vi "pcfs_dither_loop_wait_for_fifo_loop.vi"(8 "error in (no error)":errorcluster, 11 "pcfs in":refnum<class "pcfs.lvclass">) -> (0 "error out":errorcluster, 3 "pcfs out":refnum<class "pcfs.lvclass">)   [LabVIEW 2015, in "pcfs.lvclass"]
uses:
  pcfs.lvclass
  pcfs.lvclass/pcfs.ctl
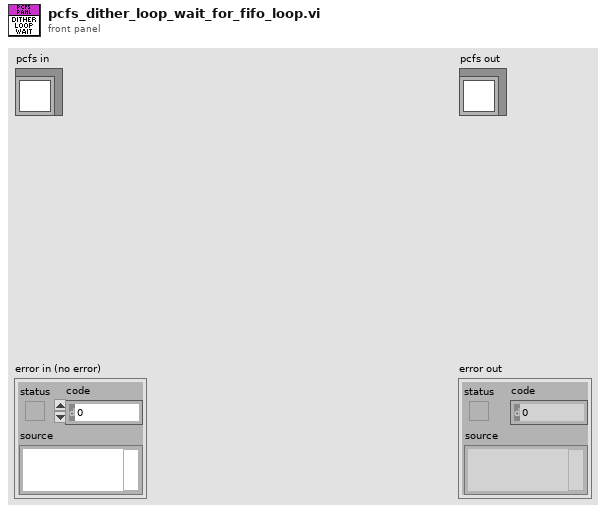
[diagram p1: front panel]
types:
  T1 = typedef "Rendezvous RefNum" = refnum<k1>
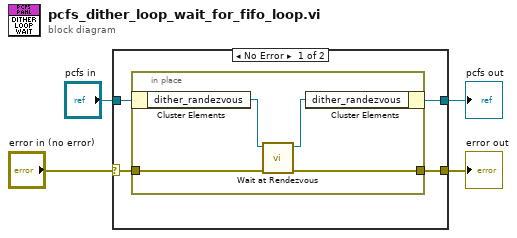
[diagram p0: block diagram]
diagram:
  n1 = case shown="No Error" "error in (no error)" {
    selector: "error in (no error)" -> [w8 w14]
    tunnel: [w5 w14] -> w3
    tunnel: [w6 w13] -> w1
    tunnel: "pcfs in" -> [w7 w13]
    frame No Error {
      n2 = in-place {
        in-place-border: w8 -> [w11]
        in-place-border: [w9] -> w5
        n3 = in-place-cluster #1(w7) -> ("dither_randezvous"=w12:T1)
        n4 = call <vilib>:"Wait at Rendezvous.vi"("error in (no error)"=w11, "rendezvous"=w12) -> ("error out"=w9:errorcluster, "rendezvous out"=w10:T1)  [unwired: 3 in, 1 out]
        n5 = in-place-cluster #1("dither_randezvous"=w10) -> (w6:refnum<class "pcfs.lvclass">)
      }
    }
    frame Error {
    }
  }
  "error out" <- w3
  "pcfs out" <- w1
